vi "DG535.set A delay.vi"(0 "i ref in":refnum<vi>, 5 "Ref Channel":string, 7 "A Delay":dbl min=0.0 max=999.999999999995 format="%.12f", 11 "error in (no error)":errorcluster) -> (4 "i ref out":refnum<vi>, 15 "error out":errorcluster)   [LabVIEW 2014, in "DG535.lvlib"]
uses:
  DG535.lvlib
panel:
  # "+"
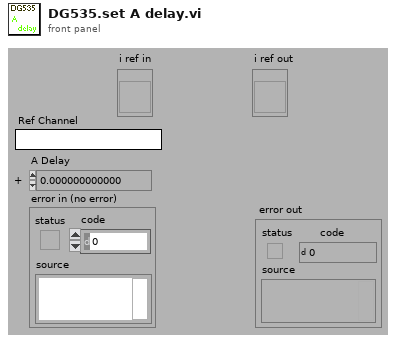
[diagram p1: front panel]
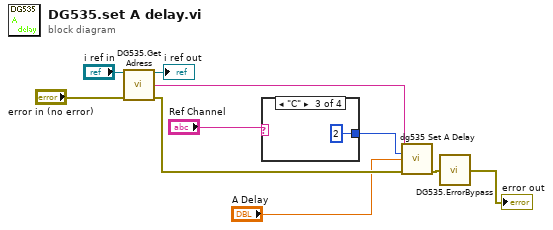
[diagram p0: block diagram]
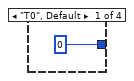
[diagram p2: hidden frame]
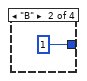
[diagram p3: hidden frame]
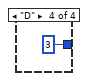
[diagram p4: hidden frame]
diagram:
  n1 = call "DG535.Get Adress.vi"("i ref in"="i ref in", "error in (no error)"="error in (no error)") -> ("i ref out"=→"i ref out":refnum<vi>, "address"=w7:string, "error out"=w6:errorcluster)  [unwired: 10 in, 1 out]
  n2 = case shown="\"C\"" "Ref Channel" {
    tunnel: [0 1 2 3] -> w2
    frame "T0", Default {
    }
    frame "B" {
    }
    frame "C" {
    }
    frame "D" {
    }
  }
  n3 = call "dg535 Set A Delay.vi"("address string"=w7, "A="=w2, "A"="A Delay", "error in"=w6) -> ("error out"=w5:errorcluster)  [unwired: 11 in]
  n4 = call "DG535.ErrorBypass.vi"("error in (no error)"=w5) -> ("error out"=→"error out":errorcluster)  [unwired: 14 in]
